vi "exclude system objects.vi"(1 "objects in":string[](array[string])) -> (0 "objects out":string[](array[string]))   [LabVIEW 2009, in "PTUtils.lvlib"]
uses:
  PTUtils.lvlib
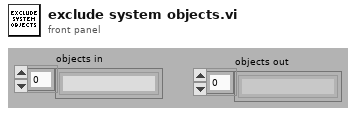
[diagram p1: front panel]
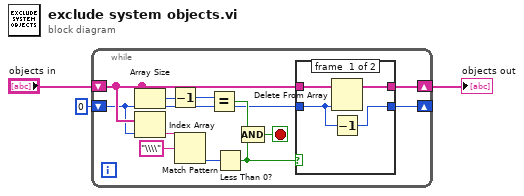
[diagram p0: block diagram]
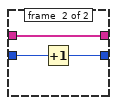
[diagram p2: hidden frame]
diagram:
  n1 = while {
    shift-right: [w9] -> _
    shift-left: 0 -> [w4]
    shift-right: [w10] -> w1
    shift-left: "objects in" -> [w11]
    stop <- w12 stop-if-true
    n2 = Array Size(array=w11) -> (size(s)=w14:i32)
    n3 = Index Array(array=w11, index=w4) -> (element=w15:string)
    n4 = Decrement(x=w14) -> (x-1=w5:i32)
    n5 = Match Pattern(string=w15, regular expression="\\\\") -> (offset past match=w7:i32)  [unwired: 1 in, 3 out]
    n6 = Equal?(x=w5, y=w4) -> (x = y?=w13:bool)
    n7 = Less Than 0?(x=w7) -> (x < 0?=w6:bool)
    n8 = Compound Arithmetic op=AND(w13, w6) -> (w12:bool)
    n9 = case shown="False" w6 {
      tunnel: w4 -> [w17 w22]
      tunnel: w11 -> [w19 w21]
      tunnel: [w18 w21] -> w10
      tunnel: [w16 w20] -> w9
      frame #0 {
        n10 = Delete From Array(array=w19, index=w17) -> (array with subset deleted=w18:string[])  [unwired: 1 in, 1 out]
        n11 = Decrement(x=w17) -> (x-1=w16:i32)
      }
      frame #1 {
        n12 = Increment(x=w22) -> (x+1=w20:i32)
      }
    }
  }
  "objects out" <- w1
